vi "Read Statistcs.vi"(8 "error in (no error)":errorcluster, 11 "CAN_RW_CORE in":refnum<class "L2ENET_RW_CORE.lvclass">) -> (0 "error out":errorcluster, 2 "Statistcs":T1, 3 "CAN_RW_CORE out":refnum<class "L2ENET_RW_CORE.lvclass">)   [LabVIEW 2021, in "L2ENET_RW_CORE.lvclass"]
uses:
  L2ENET_RW_CORE.lvclass
  L2ENET_RW_CORE.lvclass/L2ENET_RW_CORE.ctl
  typedef/Statistics.ctl
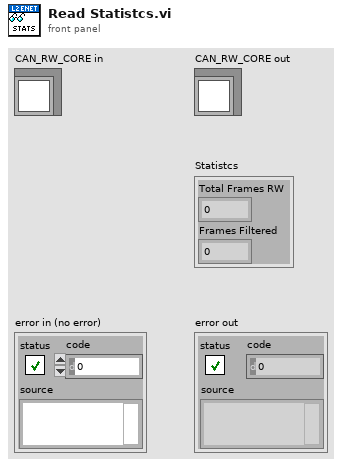
[diagram p1: front panel]
types:
  T1 = typedef "L2ENET_RW_CORE.lvclass/Statistics.ctl" = cluster{"Total Frames RW":u32, "Frames Filtered ":u32}
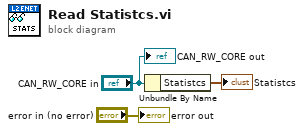
[diagram p0: block diagram]
diagram:
  n1 = Unbundle By Name("CAN_RW_CORE in") -> ("Statistcs"=→"Statistcs":T1)
  "error out" <- "error in (no error)"
  "CAN_RW_CORE out" <- "CAN_RW_CORE in"
